vi "create.exclude_id.vi"(10 "IDs":i32[](array[numeric])) -> (3 "Exclude Filter":refnum<class "exclude.lvclass">)   [LabVIEW 2020, in "nominal types.lvlib" / "channelFilter.lvlib" / "channelFilter.lvclass"]
uses:
  channelFilter.lvclass
  exclude/exclude.lvclass
  id/id.lvclass
  C:/code/labview-client/lv_src/nominal types/filterTypes/filterTypes.lvclass
  id/id.lvclass/id.ctl
  exclude/exclude.lvclass/exclude.ctl
  id/id.set.vi
  exclude/exclude.set.vi
  filterTypes/filterTypes.lvclass
  channelFilter.lvclass/channelFilter.ctl
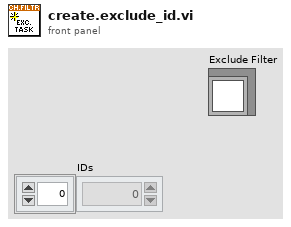
[diagram p1: front panel]
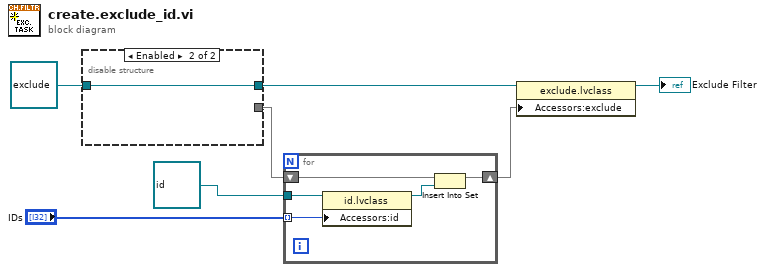
[diagram p0: block diagram]
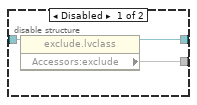
[diagram p2: hidden frame]
diagram:
  n1 = disable-structure shown="Enabled" {
    disable-tunnel: refnum<class "exclude.lvclass"> refnum ("Exclude Filter") -> [w10 w11]
    disable-tunnel: [w9 w11] -> w4
    disable-tunnel: [w8 _] -> w3
    frame Disabled {
      n2 = property class="exclude.lvclass"(reference=w10) -> (reference out=w9:refnum<class "exclude.lvclass">, "Accessors:exclude"=w8:set{refnum<class "filterTypes.lvclass">})  [unwired: 1 in, 1 out]
    }
    frame Enabled {
    }
  }
  n3 = for {
    tunnel: "IDs" -> [w16] mode=indexing
    tunnel: refnum<class "id.lvclass"> refnum ("reference") -> [w15]
    shift-right: [w12] -> w5
    shift-left: w3 -> [w14]
    n4 = property class="id.lvclass"(reference=w15, "Accessors:id"=w16) -> (reference out=w13:refnum<class "id.lvclass">)  [unwired: 1 in, 1 out]
    n5 = Insert Into Set(10:w13, 11:w14) -> (3:w12:set{refnum<class "filterTypes.lvclass">})  [unwired: 1 out]
  }
  n6 = property class="exclude.lvclass"(reference=w4, "Accessors:exclude"=w5) -> (reference out=→"Exclude Filter":refnum<class "exclude.lvclass">)  [unwired: 1 in, 1 out]
